vi "Collect.vi"(8 "error in (no error)":errorcluster, 11 "User Interface in":refnum<class "User Interface.lvclass">) -> (0 "error out":errorcluster, 3 "User Interface out":refnum<class "User Interface.lvclass">)   [LabVIEW 2017, in "DSF Core.lvlib" / "User Interface.lvclass"]
uses:
  User Interface.lvclass
  User Interface.lvclass/User Interface.ctl
  Configuration/Configuration.lvclass
  User Interface Events/User Interface Events.lvclass
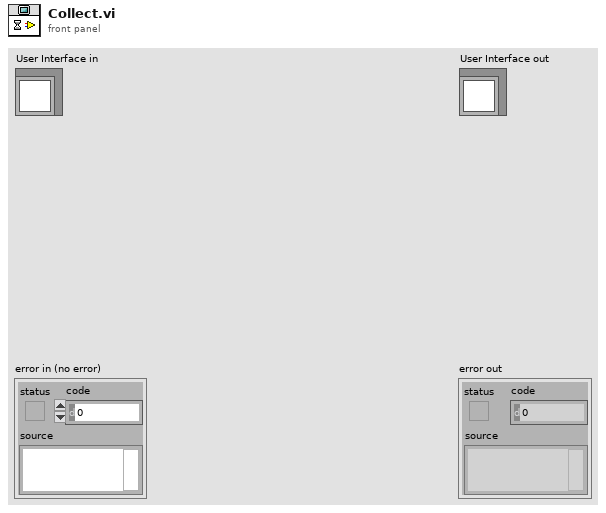
[diagram p1: front panel]
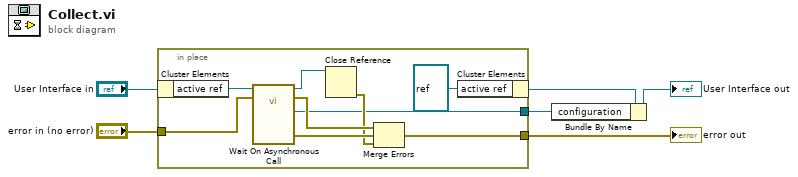
[diagram p0: block diagram]
diagram:
  n1 = in-place {
    in-place-border: [w8] -> w1
    in-place-border: [w13] -> w2
    in-place-border: "error in (no error)" -> [w12]
    n2 = in-place-cluster #1("User Interface in") -> ("active ref"=w15:refnum<vi>)
    n3 = call-by-ref "Wait On Asynchronous Call"(reference=w15, error in=w12) -> (reference out=w11:refnum<vi>, error out=w14:errorcluster, 0:"error out"=w10:errorcluster, "Configuration out"=w8:refnum<class "Configuration.lvclass">)  [unwired: 10 in]
    n4 = Close Reference(reference=w11) -> (error out=w9:errorcluster)  [unwired: 1 in]
    n5 = Merge Errors(w14, w10, w9) -> (w13:errorcluster)
    n6 = in-place-cluster #1("active ref"=refnum<vi> refnum) -> (w4:refnum<class "User Interface.lvclass">)
  }
  "error out" <- w2
  n7 = Bundle By Name(cluster=w4, "configuration"=w1) -> (→"User Interface out":refnum<class "User Interface.lvclass">)
